vi "PI_Stop_Wave_Gen.vi"(0 "System no.":i32, 11 "error in":errorcluster) -> (4 "System no. (dup)":i32, 15 "error out":errorcluster)   [LabVIEW 2009]
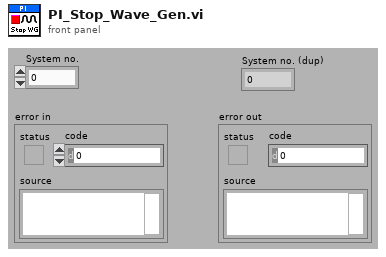
[diagram p1: front panel]
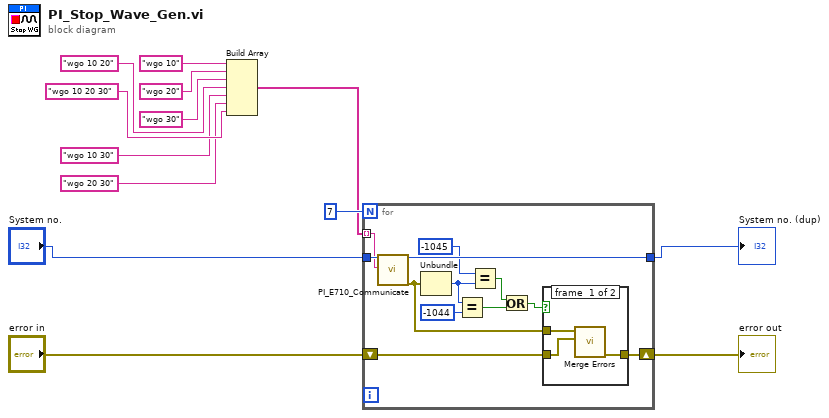
[diagram p0: block diagram]
diagram:
  n1 = Build Array("wgo 10" ("String to send"), "wgo 20" ("String to send"), "wgo 30" ("String to send"), "wgo 10 20" ("String to send"), "wgo 10 30" ("String to send"), "wgo 20 30" ("String to send"), "wgo 10 20 30" ("String to send")) -> (w12:string[])
  n2 = for {
    N: 7 -> [_]
    tunnel: "System no." -> [w25]
    tunnel: w12 -> [w24] mode=indexing
    shift-right: [w21] -> w11
    shift-left: "error in" -> [w20]
    tunnel: [w23] -> w1
    n3 = call "PI_E710_Communicate.vi"("System no."=w25, "String to send"=w24) -> ("System no. (dup)"=w23:i32, "error out"=w19:errorcluster)  [unwired: 15 in, 1 out]
    n4 = Unbundle(w19) -> ("code"=w18:i32)  [unwired: 2 out]
    n5 = Equal?(x=w18, y=-1044 ("code")) -> (x = y?=w15:bool)
    n6 = Equal?(x=-1045 ("code"), y=w18) -> (x = y?=w16:bool)
    n7 = Or(x=w16, y=w15) -> (x .or. y?=w14:bool)
    n8 = case shown="False" w14 {
      tunnel: [w28 w29] -> w21
      tunnel: w20 -> [w27 w29]
      tunnel: w19 -> [w26 _]
      frame #0 {
        n9 = call <vilib>:"Merge Errors.vi"("error in 2 (no error)"=w27, "error in 1 (no error)"=w26) -> ("error out"=w28:errorcluster)  [unwired: 5 in]
      }
      frame #1 {
      }
    }
  }
  "error out" <- w11
  "System no. (dup)" <- w1
